vi "Reroll BaseNodeType Identifiers.vi"(8 "error in":errorcluster, 11 "BaseNodeType in":refnum<k24>) -> (0 "error out":errorcluster, 3 "BaseNodeType out":refnum<k24>)   [LabVIEW 2017, in "Import Export.lvlib"]
uses:
  NationalInstruments.VeriStand.SystemStorage
  Import Export.lvlib
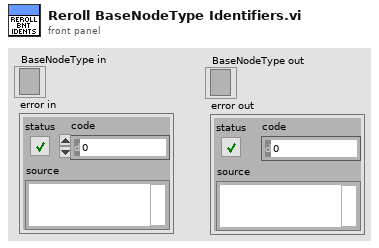
[diagram p1: front panel]
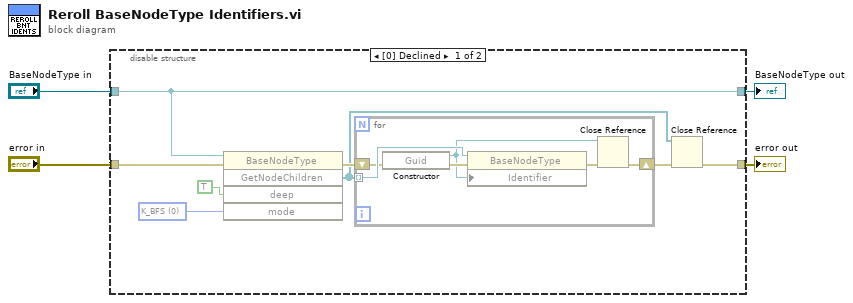
[diagram p0: block diagram]
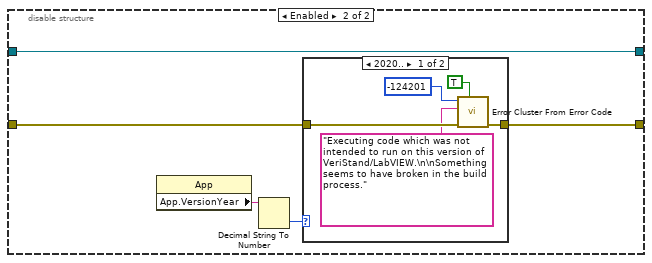
[diagram p2: hidden frame]
diagram:
  n1 = disable-structure shown="[0] Declined" {
    disable-tunnel: "BaseNodeType in" -> [w5 w19]
    disable-tunnel: "error in" -> [w7 w21]
    disable-tunnel: [w6 w20] -> w1
    disable-tunnel: [w5 w19] -> w2
    frame Disabled {
      w8 = 0 items=["K_BFS", "K_DFS", "K_CHILDONLY", "K_UP"] ("mode")
      n2 = invoke class="BaseNodeType" method="GetNodeChildren"(reference=w5, error in=w7, "deep"=TRUE, "mode"=w8) -> (error out=w12:errorcluster, "GetNodeChildren"=w11:refnum<k24>[])  [unwired: 1 in, 3 out]
      n3 = for {
        tunnel: w11 -> [w17] mode=indexing
        shift-right: [w14] -> w10
        shift-left: w12 -> [w15]
        n4 = constructor class="Guid"(error in=w15) -> (reference out=w13:refnum<k24>, error out=w18:errorcluster)  [unwired: 2 in, 1 out]
        n5 = property class="BaseNodeType"(reference=w17, error in=w18, "Identifier"=w13) -> (error out=w16:errorcluster)  [unwired: 1 out]
        n6 = Close Reference(reference=w13, error in (no error)=w16) -> (error out=w14:errorcluster)
      }
      n7 = Close Reference(reference=w11, error in (no error)=w10) -> (error out=w6:errorcluster)
    }
    frame Enabled {
      n8 = property class="App"() -> ("App.VersionYear"=w23:string)  [unwired: 2 in, 2 out]
      n9 = Decimal String To Number(string=w23) -> (number=w22:i32)  [unwired: 2 in, 1 out]
      n10 = case shown="2020.." w22 {
        tunnel: w21 -> [w26 w29]
        tunnel: [w24 w29] -> w20
        frame 2020.. {
          n11 = call <vilib>:"Error Cluster From Error Code.vi"("show call chain? (False)"=TRUE, "error in (no error)"=w26, "error message (\"\")"="Executing code which was not intended to run on this version of VeriStand/LabVIEW.\n\nSomething seems to have broken in the build process." ("error message (\"\")"), "error code (0)"=-124201) -> ("error out"=w24:errorcluster)  [unwired: 5 in]
        }
        frame ..2019 {
        }
      }
    }
  }
  "BaseNodeType out" <- w2
  "error out" <- w1
